vi "SV Multitone THD IMD SNR.vi"   [LabVIEW 2017, in "SoundVib_Multitone.lvlib"]
doc: "Performs total harmonic distortion (THD), intermodulation distortion (IMD), and signal-to-noise ratio (SNR) measurements, including measuring the fundamental tones, harmonic components, intermodulation components, and residual noise. Wire data to the <B>scaled signal [EU]</B> input to determine the polymorphic instance to use or manually select the instance."
uses:
  <vilib>/addons/Sound and Vibration/svt_Multitone Distortion/SoundVib_Multitone.lvlib
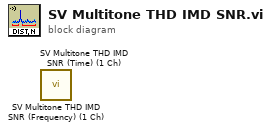
[diagram p0: block diagram]
diagram:
  n1 = call <vilib>:"SV Multitone THD IMD SNR (Frequency) (1 Ch).vi"() -> ()  [unwired: 12 in, 8 out]
  n2 = call <vilib>:"SV Multitone THD IMD SNR (Time) (1 Ch).vi"() -> ()  [unwired: 12 in, 8 out]
